vi "Parse Cluster Configuration.vi"(8 "error in (no error)":errorcluster, 10 "Cluster in":variant, 11 "Register Name in":string) -> (0 "error out":errorcluster, 2 "Cluster Configuration":T1)   [LabVIEW 2020, in "FPGA Register IO.lvlib"]
uses:
  FPGA Register IO.lvlib
  TypeDefs/Cluster Configuration.ctl
  <userlib>/_OpenG.lib/lvdata/lvdata.llb/Type Descriptor__ogtk.ctl
  <vilib>/Utility/Data Type/Type Definitions/Data Type.ctl
  TypeDefs/Cluster Configuration Store.ctl
  TypeDefs/FXP Configuration.ctl
  <vilib>/fxp/LVFixedPointRepBitsTypeDef.ctl
  <vilib>/fxp/LVFixedPointRepRangeTypeDef.ctl
  <vilib>/Utility/Data Type/NI_Data Type.lvlib
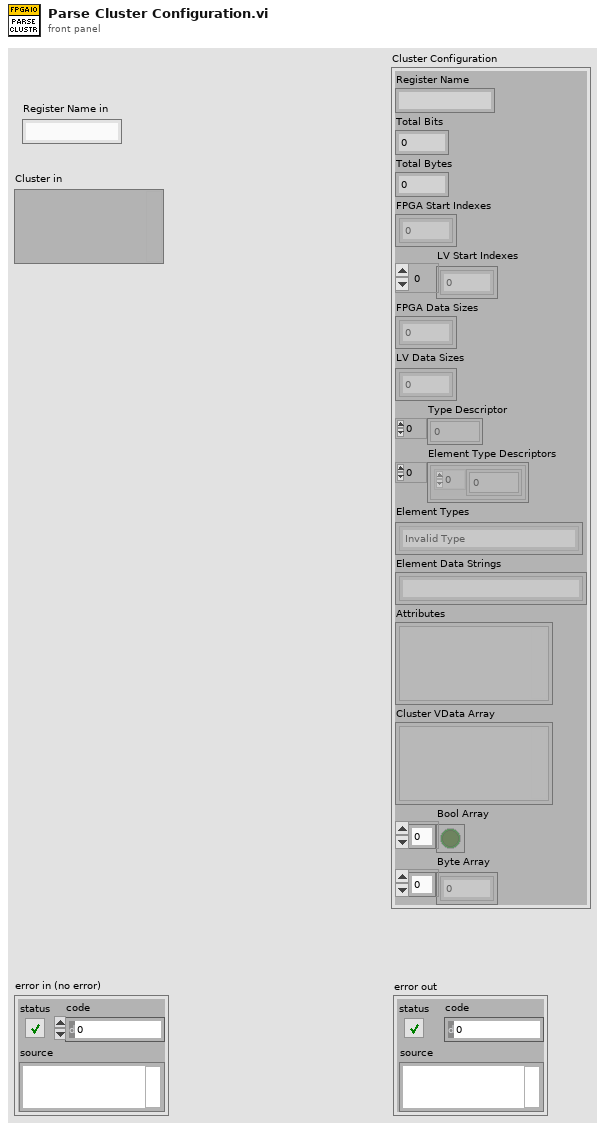
[diagram p1: front panel]
types:
  T1 = typedef "FPGA Register IO.lvlib/Cluster Configuration.ctl" = cluster{"Register Name":string, "Total Bits":i32, "Total Bytes":i32, "FPGA Start Indexes":i32[], "LV Start Indexes":i32[], "FPGA Data Sizes":i32[], "LV Data Sizes":i32[], "Type Descriptor":T2, "Element Type Descriptors":cluster{"Type Descriptor":T2}[], "Element Types":T3[], "Element Data Strings":string[], "Attributes":variant[], "Cluster VData Array":variant[], "Bool Array":bool[], "Byte Array":u8[]}
  T2 = typedef "Type Descriptor__ogtk.ctl" = i16[]
  T3 = typedef "NI_Data Type.lvlib/Data Type.ctl" = enum8{"Invalid Type", "Void", "I8", "I16", "I32", "I64", "U8", "U16", "U32", "U64", "Single Float", "Double Float", "Extended Float", "Single Complex", "Double Complex", "Extended Complex", "Enum U8", "Enum U16", "Enum U32", "Enum U64", "Single Float With Unit", "Double Float With Unit", "Extended Float With Unit", "Single Complex with Unit", "Double Complex with Unit", "Extended Complex with Unit", "Boolean", "String", "Path", "Picture", "Tag", "Array", "Cluster", "Variant", "LV Variant", "Waveform", "Timestamp", "Digital Waveform", "Digital Data", "ExpressData", "Refnum", "External Data", "VI", "Poly VI", "LabVIEW Class Instance", "Fixed Point", "Set Collection", "Map Collection"}
  T4 = typedef "FPGA Register IO.lvlib/Cluster Configuration Store.ctl" = cluster{"Register Names":string[], "Cluster Configurations":T1[]}
  T5 = typedef "FPGA Register IO.lvlib/FXP Configuration.ctl" = cluster{"FXP Representation":T6, "FXP Range":T7}
  T6 = typedef "LVFixedPointRepBitsTypeDef.ctl" = cluster{"Signed":bool, "Word Length":u32, "Integer Word Length":i32}
  T7 = typedef "LVFixedPointRepRangeTypeDef.ctl" = cluster{"Range Min":dbl, "Range Max":dbl, "Delta":dbl}
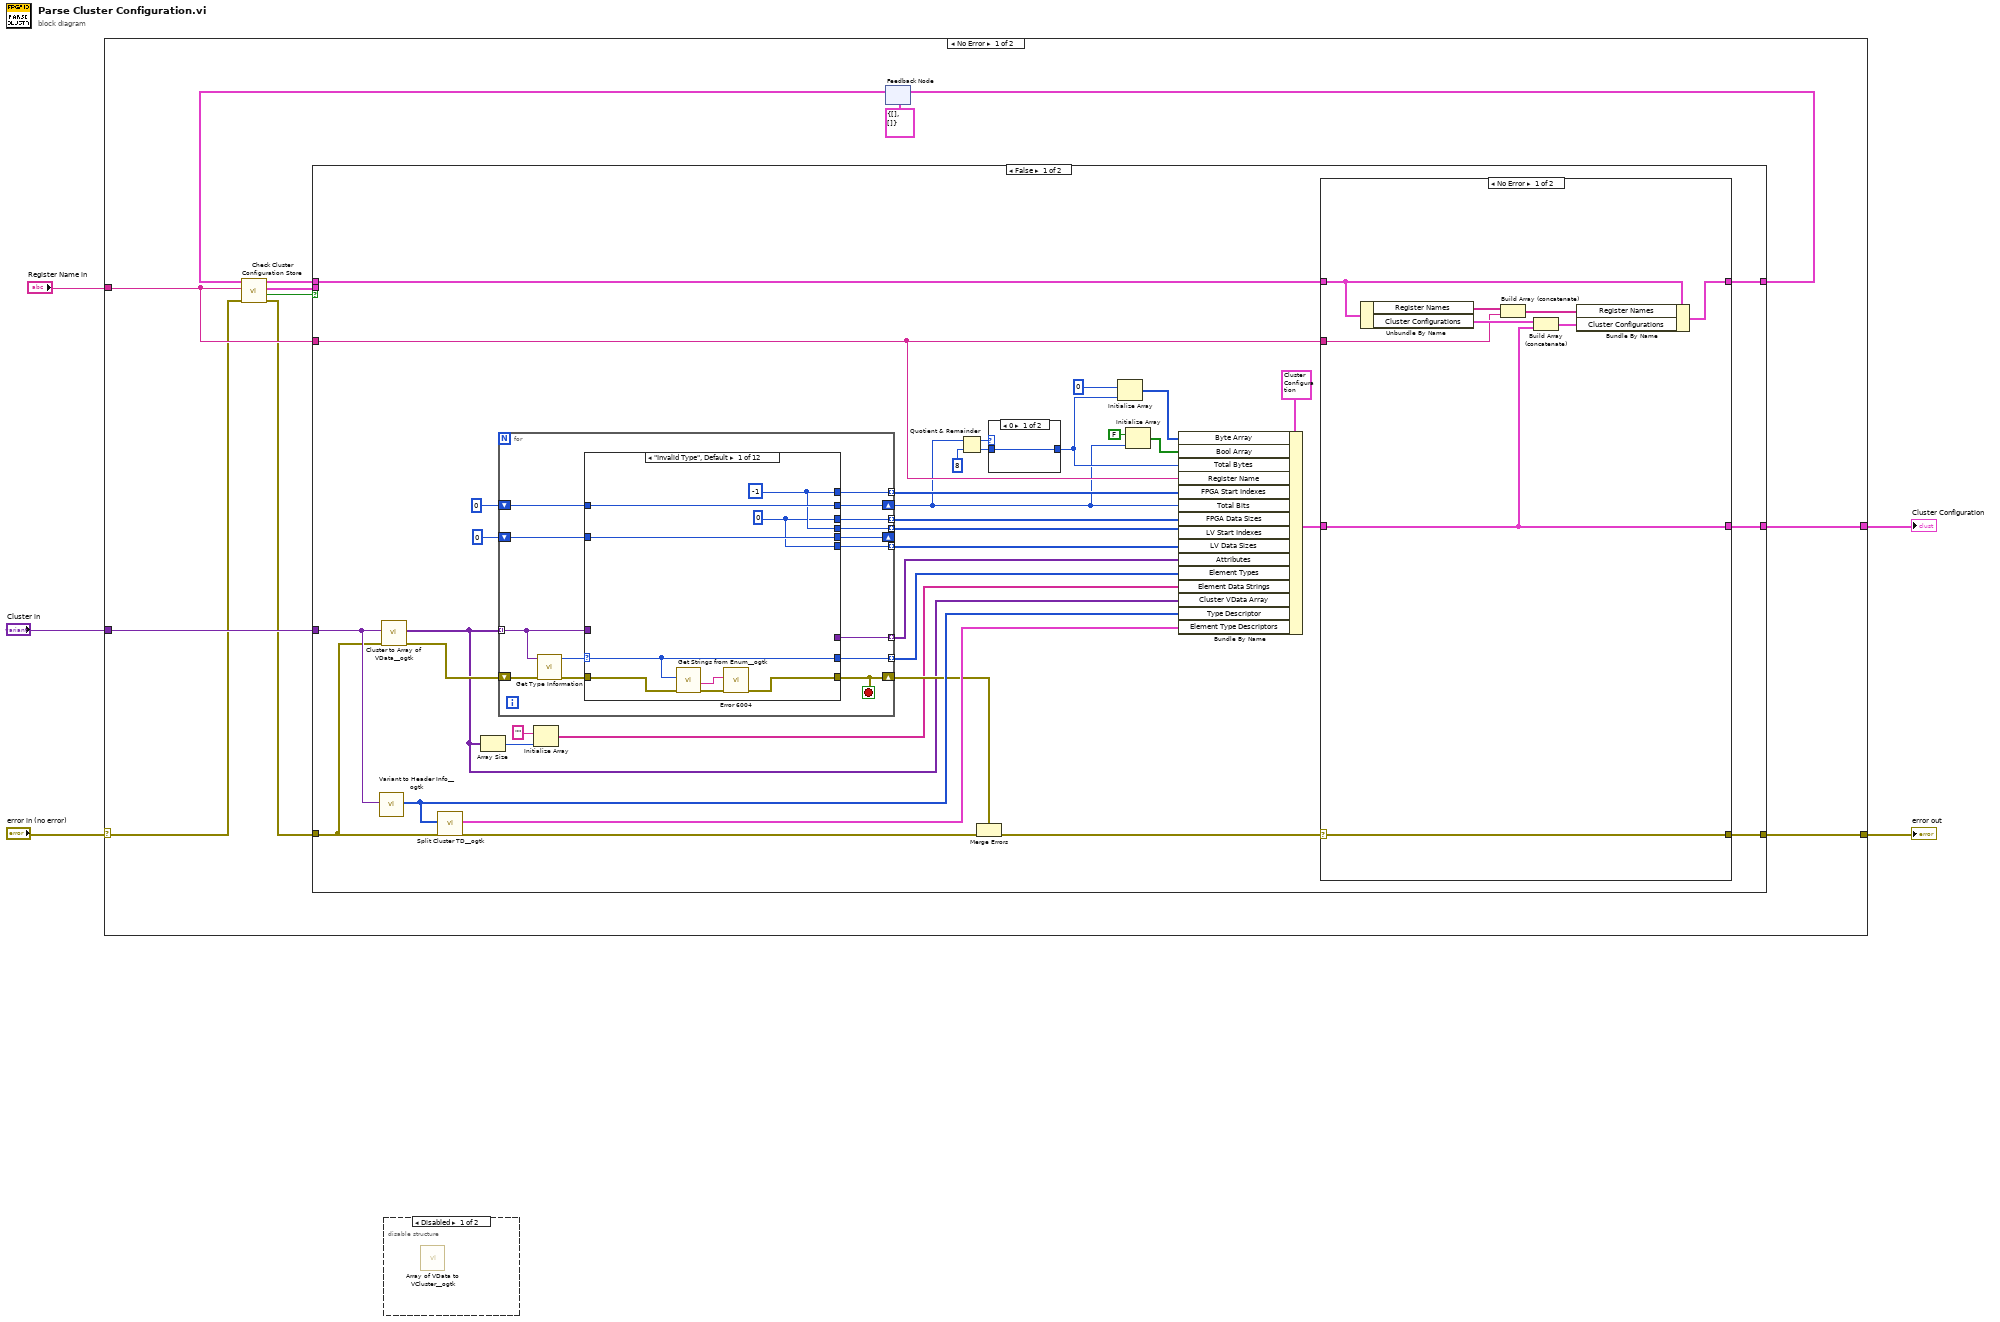
[diagram p0: block diagram]
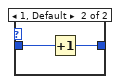
[diagram p2: hidden frame]
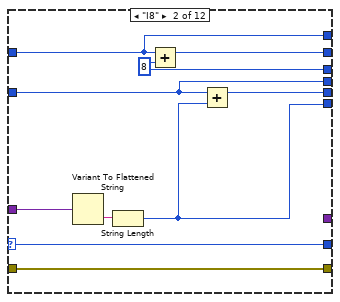
[diagram p4: hidden frame]
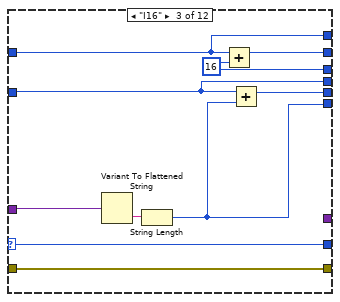
[diagram p5: hidden frame]
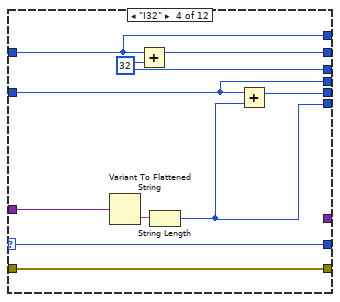
[diagram p6: hidden frame]
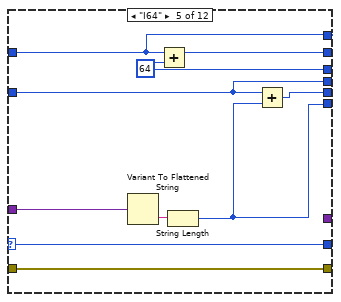
[diagram p7: hidden frame]
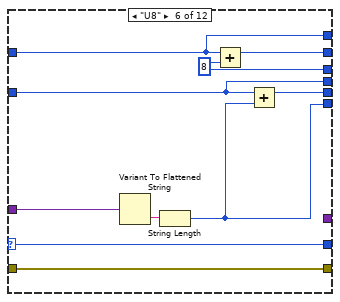
[diagram p8: hidden frame]
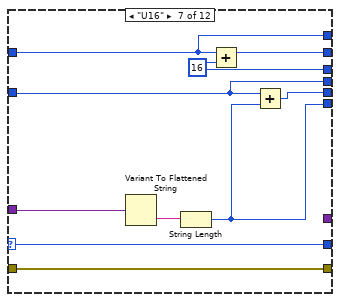
[diagram p9: hidden frame]
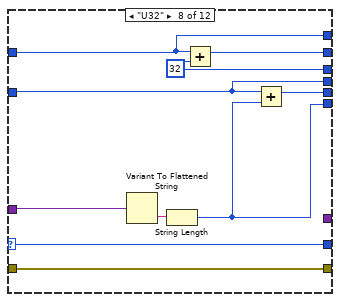
[diagram p10: hidden frame]
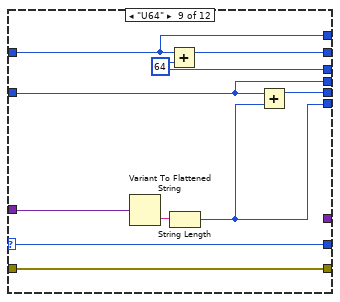
[diagram p11: hidden frame]
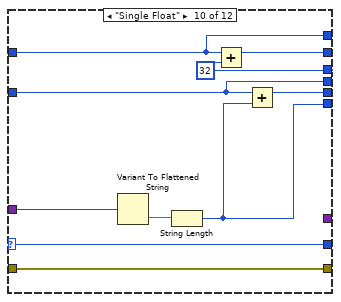
[diagram p12: hidden frame]
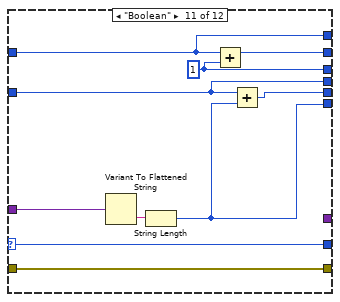
[diagram p13: hidden frame]
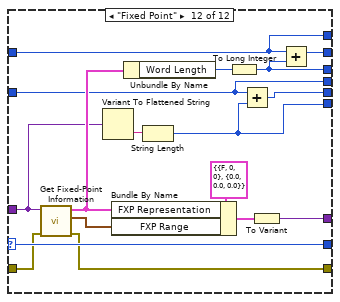
[diagram p14: hidden frame]
diagram:
  n1 = case shown="No Error" "error in (no error)" {
    selector: "error in (no error)" -> [w7 w213]
    tunnel: "Cluster in" -> [w16 _]
    tunnel: [w17 w213] -> w3
    tunnel: "Register Name in" -> [w13 _]
    tunnel: [w8 _] -> w1
    frame No Error {
      n2 = feedback #1(T4 {"Register Names"=[], "Cluster Configurations"=[]} ("Cluster Configuration Store out")) -> (w11:T4)
      n3 = call "Check Cluster Configuration Store.vi"("error in (no error)"=w7, "register name"=w13, "Cluster Configuration Store in"=w11) -> ("error IO"=w6:errorcluster, "Found"=w15:bool, "Cluster Configuration out"=w10:T1, "Cluster Configuration Store out"=w14:T4)  [unwired: 5 in]
      n4 = case shown="False" w15 {
        tunnel: w16 -> [w42 _]
        tunnel: w6 -> [w39 w212]
        tunnel: [w48 w212] -> w17
        tunnel: w14 -> [w46 w211]
        tunnel: w13 -> [w27 _]
        tunnel: [w45 w211] -> w12
        tunnel: w10 -> [_ w210]
        tunnel: [w44 w210] -> w8
        frame False {
          n5 = call <userlib>:"Variant to Header Info__ogtk.vi"("Variant"=w42) -> ("Type Descriptor"=w41:T2)  [unwired: 3 in, 2 out]
          n6 = call <userlib>:"Cluster to Array of VData__ogtk.vi"("error in (no error)"=w39, "Cluster"=w42) -> ("error out"=w43:errorcluster, "Array of VData"=w34:variant[])  [unwired: 8 in]
          n7 = call <userlib>:"Split Cluster TD__ogtk.vi"("error in (no error)"=w39, "Type Descriptor"=w41) -> ("error out"=w38:errorcluster, "Type Descriptors"=w40:cluster{"Type Descriptor":T2}[])  [unwired: 8 in]
          n8 = Array Size(array=w34) -> (size(s)=w35:i32)
          n9 = for {
            tunnel: w34 -> [w82] mode=indexing
            shift-right: [w80] -> w18
            shift-left: 0 -> [w81]
            tunnel: [w79] -> w49 mode=indexing
            tunnel: [w78] -> w50 mode=indexing
            tunnel: [w77] -> w51 mode=indexing
            tunnel: [w76] -> w31 mode=indexing
            shift-right: [w73] -> w37
            shift-left: w43 -> [w75]
            tunnel: [w72] -> w30 mode=indexing
            shift-right: [w70] -> _
            shift-left: 0 -> [w71]
            tunnel: [w69] -> w28 mode=indexing
            stop <- w73 stop-if-true
            n10 = call <vilib>:"Get Type Information.vi"("error in (no error)"=w75, "variant"=w82) -> ("error out"=w74:errorcluster, "type"=w83:T3)  [unwired: 5 in, 3 out]
            n11 = case shown="\"Invalid Type\", Default" w83 {
              selector: w83 -> [w89 w100 w110 w120 w130 w140 w150 w160 w170 w180 w190 w206]
              tunnel: w82 -> [_ w96 w106 w116 w126 w136 w146 w156 w166 w176 w186 w196]
              tunnel: w81 -> [w92 w101 w111 w121 w131 w141 w151 w161 w171 w181 w191 w207]
              tunnel: [w92 w102 w112 w122 w132 w142 w152 w162 w172 w182 w192 w208] -> w80
              tunnel: [w86 w101 w111 w121 w131 w141 w151 w161 w171 w181 w191 w207] -> w79
              tunnel: [w89 w100 w110 w120 w130 w140 w150 w160 w170 w180 w190 w206] -> w78
              tunnel: [w84 w99 w109 w119 w128 w139 w149 w159 w169 w179 w189 w205] -> w77
              tunnel: [_ _ _ _ _ _ _ _ _ _ _ w200] -> w76
              tunnel: w74 -> [w88 w98 w108 w118 w129 w138 w148 w158 w168 w178 w188 w199]
              tunnel: [w87 w98 w108 w118 w129 w138 w148 w158 w168 w178 w188 w198] -> w73
              tunnel: [w84 w95 w103 w115 w124 w135 w145 w154 w164 w173 w183 w194] -> w72
              tunnel: w71 -> [w85 w93 w105 w113 w123 w133 w143 w153 w163 w174 w184 w193]
              tunnel: [w85 w94 w104 w114 w125 w134 w144 w155 w165 w175 w185 w195] -> w70
              tunnel: [w86 w93 w105 w113 w123 w133 w143 w153 w163 w174 w184 w193] -> w69
              frame "Invalid Type", Default {
                w84 = 0 ("y")
                w86 = -1
                n12 = call <userlib>:"Get Strings from Enum__ogtk.vi"("error in (no error)"=w88, "Enum"=w89) -> ("error out"=w90:errorcluster, "String Value"=w91:string)  [unwired: 6 in, 2 out]
                n13 = call "Error 6004.vi"("error in (no error)"=w90, "datatype"=w91) -> ("error out"=w87:errorcluster)  [unwired: 9 in]
              }
              frame "I8" {
                w99 = 8 ("y")
                n14 = Variant To Flattened String(Variant=w96) -> (data string=w97:string)  [unwired: 1 out]
                n15 = String Length(string=w97) -> (length=w95:i32)
                n16 = Add(x=w101, y=w99) -> (x+y=w102:i32)
                n17 = Add(x=w93, y=w95) -> (x+y=w94:i32)
              }
              frame "I16" {
                w109 = 16 ("y")
                n18 = Variant To Flattened String(Variant=w106) -> (data string=w107:string)  [unwired: 1 out]
                n19 = String Length(string=w107) -> (length=w103:i32)
                n20 = Add(x=w111, y=w109) -> (x+y=w112:i32)
                n21 = Add(x=w105, y=w103) -> (x+y=w104:i32)
              }
              frame "I32" {
                w119 = 32 ("y")
                n22 = Variant To Flattened String(Variant=w116) -> (data string=w117:string)  [unwired: 1 out]
                n23 = Add(x=w121, y=w119) -> (x+y=w122:i32)
                n24 = String Length(string=w117) -> (length=w115:i32)
                n25 = Add(x=w113, y=w115) -> (x+y=w114:i32)
              }
              frame "I64" {
                w128 = 64 ("y")
                n26 = Variant To Flattened String(Variant=w126) -> (data string=w127:string)  [unwired: 1 out]
                n27 = Add(x=w131, y=w128) -> (x+y=w132:i32)
                n28 = String Length(string=w127) -> (length=w124:i32)
                n29 = Add(x=w123, y=w124) -> (x+y=w125:i32)
              }
              frame "U8" {
                w139 = 8 ("y")
                n30 = Variant To Flattened String(Variant=w136) -> (data string=w137:string)  [unwired: 1 out]
                n31 = String Length(string=w137) -> (length=w135:i32)
                n32 = Add(x=w141, y=w139) -> (x+y=w142:i32)
                n33 = Add(x=w133, y=w135) -> (x+y=w134:i32)
              }
              frame "U16" {
                w149 = 16 ("y")
                n34 = Variant To Flattened String(Variant=w146) -> (data string=w147:string)  [unwired: 1 out]
                n35 = String Length(string=w147) -> (length=w145:i32)
                n36 = Add(x=w151, y=w149) -> (x+y=w152:i32)
                n37 = Add(x=w143, y=w145) -> (x+y=w144:i32)
              }
              frame "U32" {
                w159 = 32 ("y")
                n38 = Variant To Flattened String(Variant=w156) -> (data string=w157:string)  [unwired: 1 out]
                n39 = String Length(string=w157) -> (length=w154:i32)
                n40 = Add(x=w161, y=w159) -> (x+y=w162:i32)
                n41 = Add(x=w153, y=w154) -> (x+y=w155:i32)
              }
              frame "U64" {
                w169 = 64 ("y")
                n42 = Variant To Flattened String(Variant=w166) -> (data string=w167:string)  [unwired: 1 out]
                n43 = Add(x=w171, y=w169) -> (x+y=w172:i32)
                n44 = String Length(string=w167) -> (length=w164:i32)
                n45 = Add(x=w163, y=w164) -> (x+y=w165:i32)
              }
              frame "Single Float" {
                w179 = 32 ("y")
                n46 = Variant To Flattened String(Variant=w176) -> (data string=w177:string)  [unwired: 1 out]
                n47 = String Length(string=w177) -> (length=w173:i32)
                n48 = Add(x=w181, y=w179) -> (x+y=w182:i32)
                n49 = Add(x=w174, y=w173) -> (x+y=w175:i32)
              }
              frame "Boolean" {
                w189 = 1 ("y")
                n50 = Variant To Flattened String(Variant=w186) -> (data string=w187:string)  [unwired: 1 out]
                n51 = String Length(string=w187) -> (length=w183:i32)
                n52 = Add(x=w191, y=w189) -> (x+y=w192:i32)
                n53 = Add(x=w184, y=w183) -> (x+y=w185:i32)
              }
              frame "Fixed Point" {
                n54 = call <vilib>:"Get Fixed-Point Information.vi"("error in (no error)"=w199, "variant"=w196) -> ("error out"=w198:errorcluster, "FXP range"=w203:T7, "FXP representation"=w202:T6)  [unwired: 6 in, 1 out]
                n55 = Variant To Flattened String(Variant=w196) -> (data string=w197:string)  [unwired: 1 out]
                n56 = Bundle By Name(cluster=T5 {"FXP Representation"={"Signed"=FALSE, "Word Length"=0, "Integer Word Length"=0}, "FXP Range"={"Range Min"=0.0, "Range Max"=0.0, "Delta"=0.0}} ("FXP Configuration"), "FXP Representation"=w202, "FXP Range"=w203) -> (w201:T5)
                n57 = Unbundle By Name(w202) -> ("Word Length"=w209:u32)
                n58 = String Length(string=w197) -> (length=w194:i32)
                n59 = To Long Integer(number=w209) -> (32bit integer=w205:i32)
                n60 = Add(x=w193, y=w194) -> (x+y=w195:i32)
                n61 = To Variant(anything=w201) -> (Variant=w200:variant)
                n62 = Add(x=w207, y=w205) -> (x+y=w208:i32)
              }
            }
          }
          n63 = Initialize Array("" ("String"), w35) -> (w32:string[])
          n64 = Quotient & Remainder(x=w18, y=8) -> (x-y*floor(x/y)=w25:i32, floor(x/y)=w26:i32)
          n65 = Merge Errors(w37, w38) -> (w36:errorcluster)
          n66 = case shown="0" w25 {
            tunnel: w26 -> [w54 w56]
            tunnel: [w54 w55] -> w19
            frame 0 {
            }
            frame 1, Default {
              n67 = Increment(x=w56) -> (x+1=w55:i32)
            }
          }
          n68 = Initialize Array(u8 0 ("y"), w19) -> (w22:u8[])
          n69 = Initialize Array(FALSE ("Boolean"), w18) -> (w20:bool[])
          n70 = Bundle By Name(cluster=T1 {"Register Name"="", "Total Bits"=0, "Total Bytes"=0, "FPGA Start Indexes"=[], "LV Start Indexes"=[], "FPGA Data Sizes"=[], "LV Data Sizes"=[], "Type Descriptor"=[], "Element Type Descriptors"=[], "Element Types"=[], "Element Data Strings"=[], "Attributes"=[], "Cluster VData Array"=[], "Bool Array"=[], "Byte Array"=[]} ("Cluster Configuration"), "Byte Array"=w22, "Bool Array"=w20, "Total Bytes"=w19, "Register Name"=w27, "FPGA Start Indexes"=w49, "Total Bits"=w18, "FPGA Data Sizes"=w51, "LV Start Indexes"=w28, "LV Data Sizes"=w30, "Attributes"=w31, "Element Types"=w50, "Element Data Strings"=w32, "Cluster VData Array"=w34, "Type Descriptor"=w41, "Element Type Descriptors"=w40) -> (w47:T1)
          n71 = case shown="No Error" w36 {
            selector: w36 -> [w65 w68]
            tunnel: [w65 w68] -> w48
            tunnel: w47 -> [w57 w66]
            tunnel: w46 -> [w61 w67]
            tunnel: w27 -> [w62 _]
            tunnel: [w58 w67] -> w45
            tunnel: [w57 w66] -> w44
            frame No Error {
              n72 = Unbundle By Name(w61) -> ("Register Names"=w64:string[], "Cluster Configurations"=w63:T1[])
              n73 = Build Array (concatenate)(w64, w62) -> (w60:string[])
              n74 = Build Array (concatenate)(w63, w57) -> (w59:T1[])
              n75 = Bundle By Name(cluster=w61, "Register Names"=w60, "Cluster Configurations"=w59) -> (w58:T4)
            }
            frame Error {
            }
          }
        }
        frame True {
        }
      }
      n76 = feedback-in #1(w12) -> ()
    }
    frame Error {
    }
  }
  "Cluster Configuration" <- w1
  "error out" <- w3
  n77 = disable-structure shown="Disabled" {
    frame Disabled {
      n78 = call <userlib>:"Array of VData to VCluster__ogtk.vi"() -> ()  [unwired: 10 in, 2 out]
    }
    frame Enabled {
    }
  }
